vi "GetTemplatePath.vi"(0 "LibWriter":refnum<class "LibWriter.lvclass">, 1 "LibTemplateSubDirectory":string, 5 "error in (no error)":errorcluster) -> (14 "LibWriter":refnum<class "LibWriter.lvclass">, 15 "FolderPathOut":path, 17 "MethodTemplatePathOut":path, 18 "TemplateSettings":T1, 19 "error out":errorcluster)   [LabVIEW 2014, in "LibWriter.lvclass"]
uses:
  <resource>/Framework/Providers/Open_GDS/ClassProviders/LibProvider_BaseClassInterface/LibWriter_class/ClassWriter_class/LibWriter.lvclass
  <resource>/Framework/Providers/Open_GDS/ClassProviders/LibProvider_BaseClassInterface/LibWriter_class/ClassWriter_class/TemplateSettings.ctl
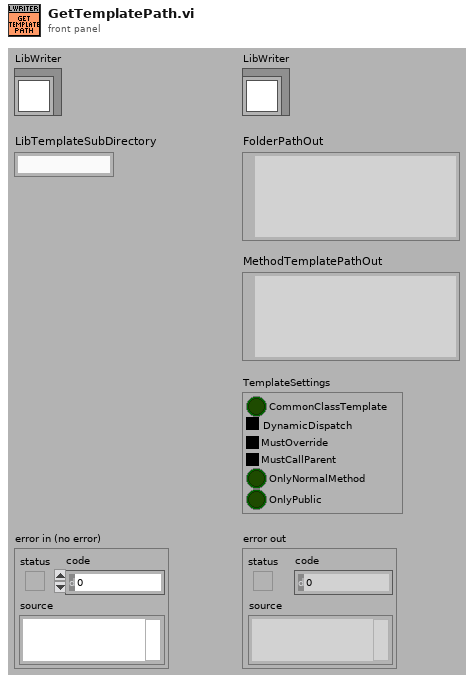
[diagram p1: front panel]
types:
  T1 = typedef "LibWriter.lvclass/TemplateSettings.ctl" = cluster{"CommonClassTemplate":bool, "DynamicDispatch":enum8{"False", "True", "Mixed"}, "MustOverride":enum8{"False", "True", "Mixed"}, "MustCallParent":enum8{"False", "True", "Mixed"}, "OnlyNormalMethod":bool, "OnlyPublic":bool}
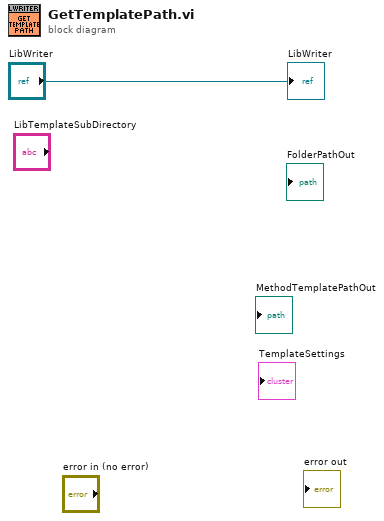
[diagram p0: block diagram]
diagram:
  "LibWriter" <- "LibWriter"
